vi "_Remote Update DAC Channels.vi"(2 "In DAC(F)":bool, 3 "UserValue":dbl[](array[numeric]), 4 "Ch#":i32[](array[numeric])) -> (1 "DACValue":i32[](array[numeric]))   [LabVIEW 2012]
uses:
  Type/_RT Active Ch.ctl
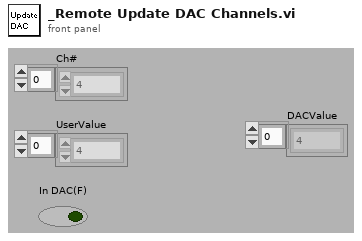
[diagram p1: front panel]
types:
  T1 = typedef "_RT Active Ch.ctl" = cluster{"Start":i32, "Step":i32, "ChID":i32}
  T2 = typedef "_RT Configuration 2.ctl" = cluster{"Name":string, "Ch#":u8, "Min":dbl, "Max":dbl, "Def+":dbl, "Def-":dbl, "Offset":dbl, "Slope":dbl, "Type":u8, "Description":string, "SettleT":dbl}
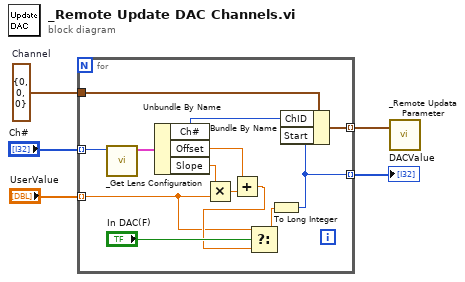
[diagram p0: block diagram]
diagram:
  w3 = T1 {"Start"=0, "Step"=0, "ChID"=0}  # Channel
  n1 = for {
    tunnel: "Ch#" -> [w14] mode=indexing
    tunnel: "UserValue" -> [w9] mode=indexing
    tunnel: w3 -> [w13]
    tunnel: [w7] -> w2 mode=indexing
    tunnel: [w12] -> w1 mode=indexing
    n2 = call "_Get Lens Configuration.vi"("Channel #"=w14) -> ("Lens Configuration"=w18:T2)  [unwired: 1 in, 5 out]
    n3 = Unbundle By Name(w18) -> ("Ch#"=w6:u8, "Offset"=w15:dbl, "Slope"=w17:dbl)
    n4 = Multiply(x=w17, y=w9) -> (x*y=w16:dbl)
    n5 = Add(x=w15, y=w16) -> (x+y=w10:dbl)
    n6 = Select(t=w9, s="In DAC(F)", f=w10) -> (s? t:f=w8:dbl)
    n7 = To Long Integer(number=w8) -> (32bit integer=w7:i32)
    n8 = Bundle By Name(cluster=w13, "ChID"=w6, "Start"=w7) -> (w12:T1)
  }
  "DACValue" <- w2
  n9 = call "_Remote Updata Parameter.vi"("Parameters"=w1) -> ()  [unwired: 1 in, 1 out]
